vi "Actor Core.vi"(8 "error in":errorcluster, 11 "Post Analysis in":refnum<class "Post Analysis.lvclass">) -> (0 "error out":errorcluster, 3 "Actor out":refnum<class "Actor.lvclass">)   [LabVIEW 2023, in "Data Analysis.lvlib" / "Post Analysis.lvlib" / "Post Analysis.lvclass"]
doc: "(<B>Filename</B>: Actor Framework.lvlib:Actor.lvclass:Actor Core.vi)\n\nReceives messages to the actor, reacts to them, and initiates any error handling that may shut the actor down.\n\nDescendant classes may override this VI to append parallel tasks for the actor to complete while it handles messages. Overrides use the Call Parent Class Method node."
uses:
  Post Analysis.lvclass
  Post Analysis.lvclass/Post Analysis.ctl
  <vilib>/ActorFramework/Actor/Actor.lvclass
  Post Analysis Messages/Init App Msg/Init App Msg.lvclass
  Subpanel-Abstract Messages/Close SP Msg/Close SP Msg.lvclass
  Post Analysis Messages/Launcher Nested Actor Caller Msg/Launcher Nested Actor Caller Msg.lvclass
  Post Analysis Messages/Test Schema Selector Update Msg/Test Schema Selector Update Msg.lvclass
  Post Analysis Messages/Report Data Update the Caller Msg/Report Data Update the Caller Msg.lvclass
  Control/Report.ctl
  Data Analysis.lvlib
  Post Analysis Messages/Filter Name Update the Selector Msg/Filter Name Update the Selector Msg.lvclass
  Post Analysis Messages/Filter Data Clear Msg/Filter Data Clear Msg.lvclass
  Post Analysis Messages/Update Test Schema Msg/Update Test Schema Msg.lvclass
  Post Analysis Messages/Delete the Schema Msg/Delete the Schema Msg.lvclass
  C:/Program Files/National Instruments/LabVIEW 2023/vi.lib/ActorFramework/Actor/Actor.lvclass
  Control/SideMenuBar.ctl
panel:
  in  "Test Phase":string(combo)
  in  "Product":string(combo)
  in  "Test Name":string(combo)
  in  "Delete Log":bool
  in  "Refresh Schema":bool
  in  "Reset Filter":bool
  in  "Test Mode":string(combo)
  in  "Stop Test Cycle":string(combo) caption="Test Cycle"
  in  "Start Test Cycle":string(combo) caption="Test Cycle"
  in  "Test Socket":string(combo)
  in  "Frame Type":string(combo)="fe_frame_log"
  in  "Log in And Out":bool
  in  "Menubar":T1(radio)
  in  "Stop":bool
  out "User":string="Coder "
  in  "Menu":bool
  out "Time":string="03:22:21 PM"
  out "Date":string="18/02/2019"
  out "User Level":string="Operator"
  out "Panel Name":string="Test Panel"
  in  "Sidebar":T2
  in  "Test Log":string(combo)
  # "LTT DATA ANALYSER"
  # "to"
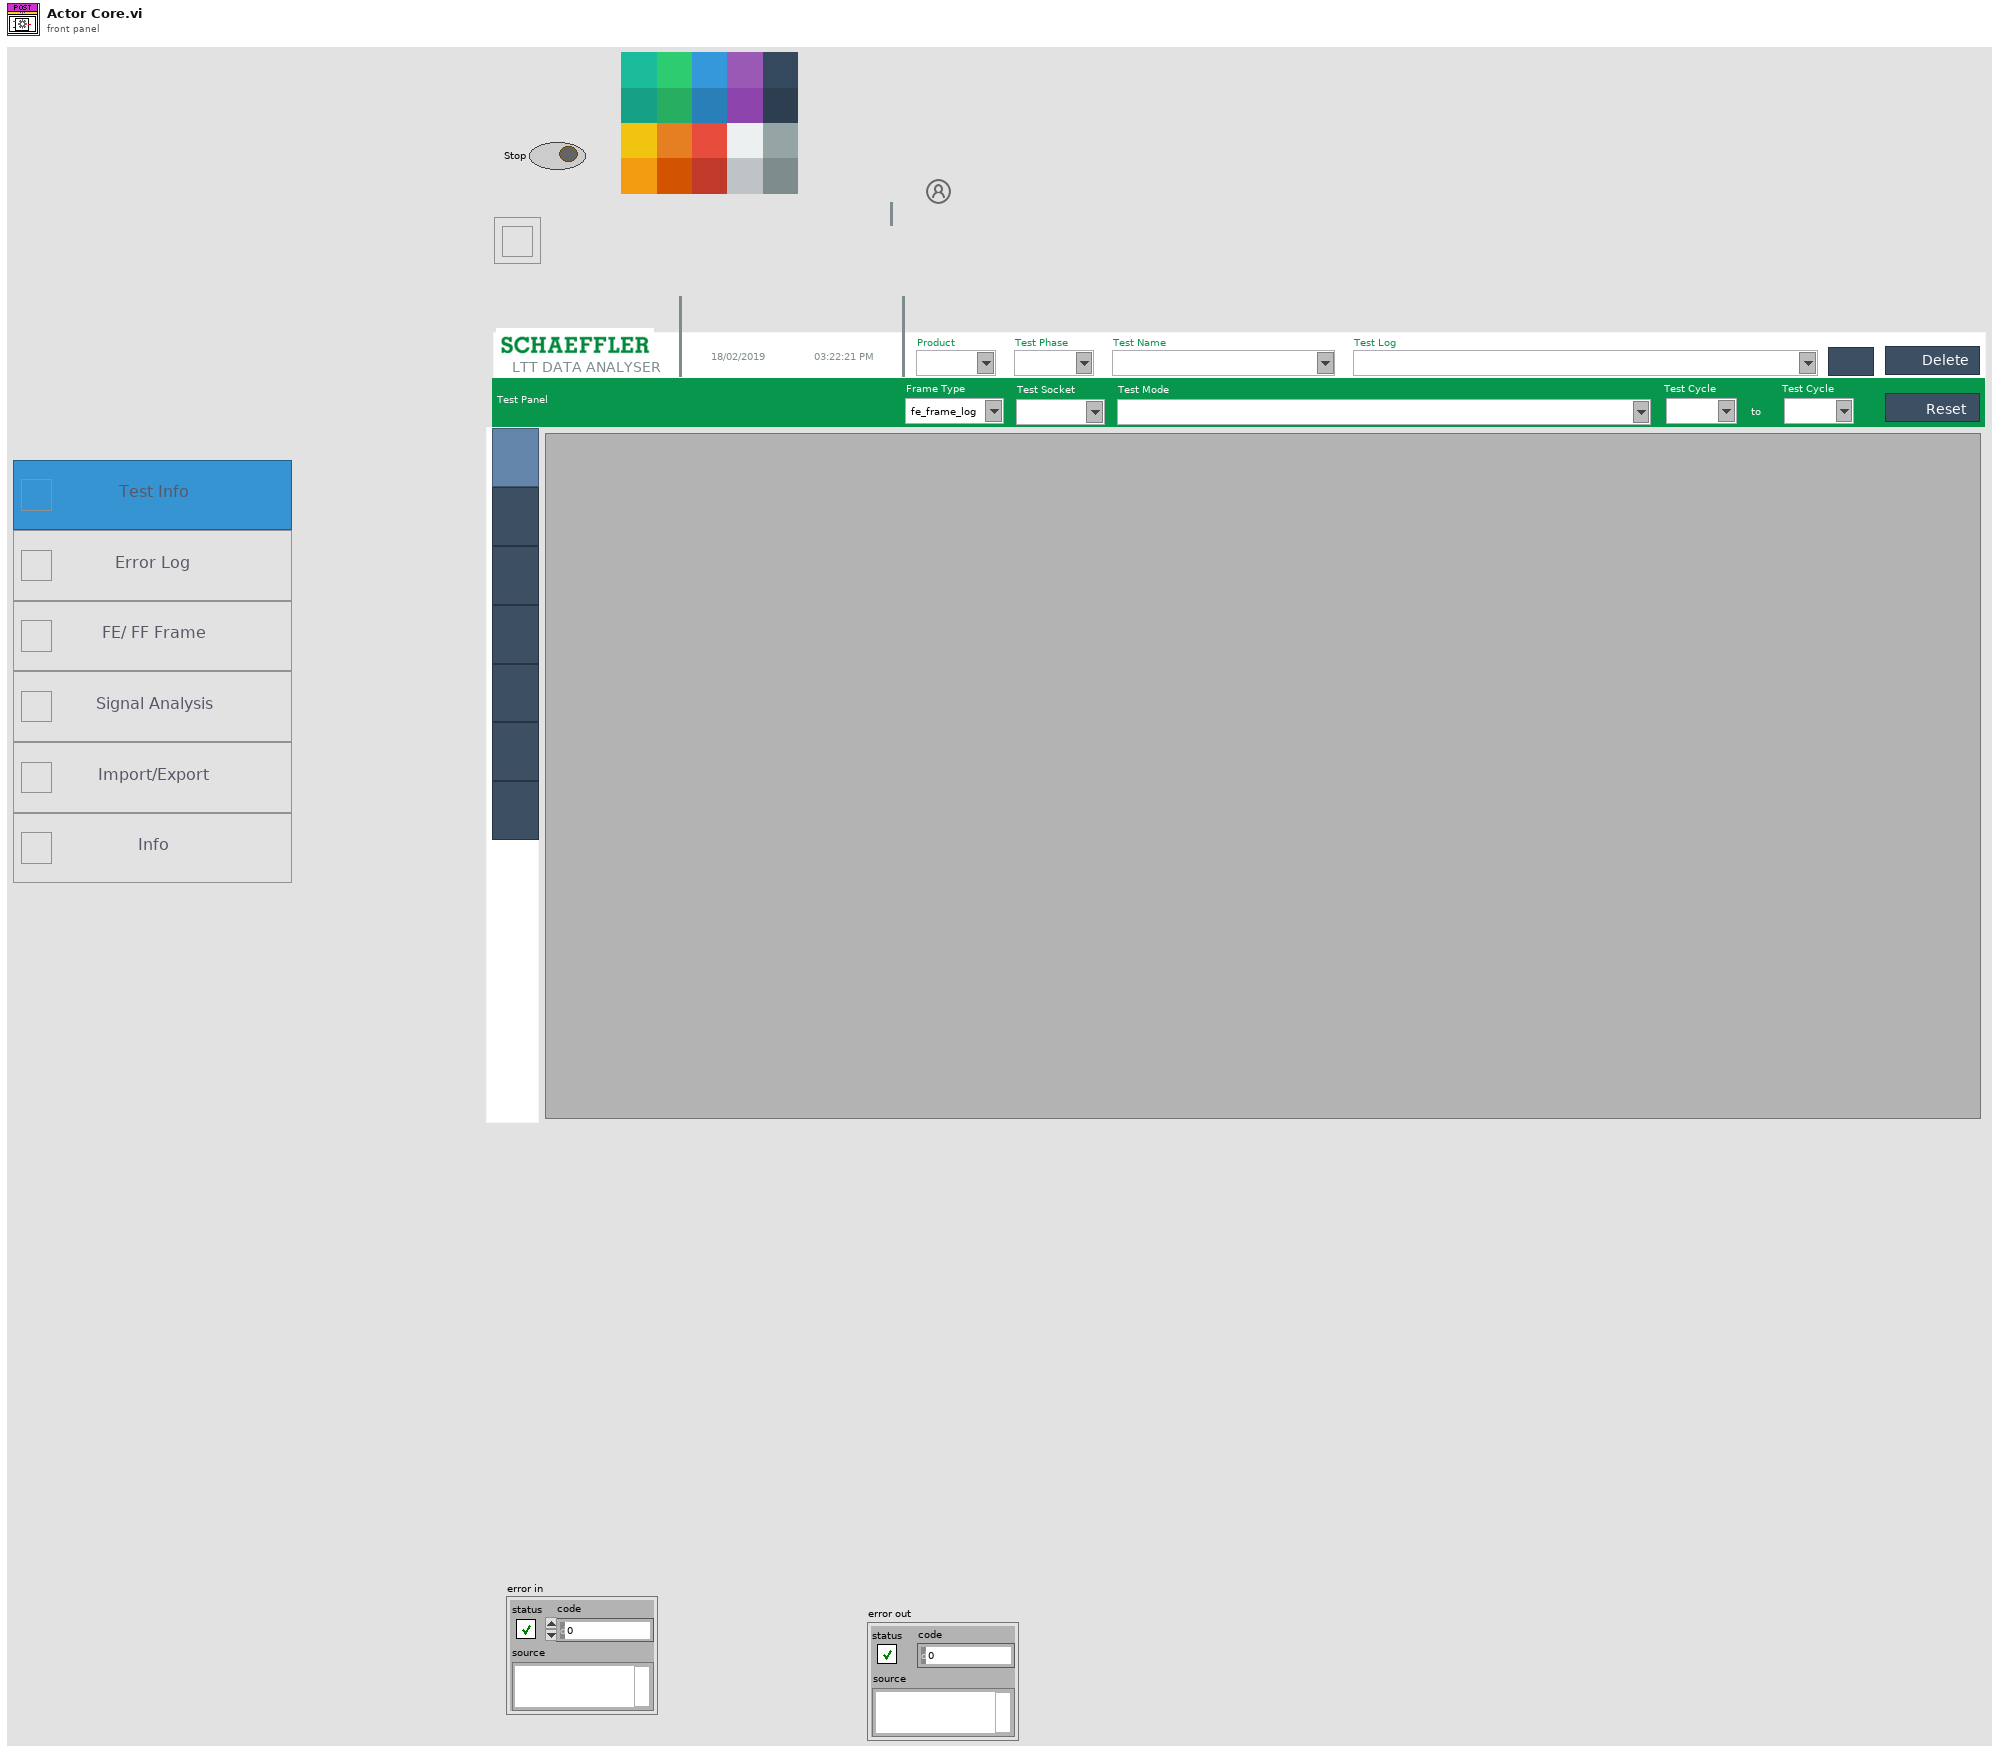
[diagram p1: front panel]
types:
  T1 = enum32{"Test Info", "Error Log", "FE/ FF Frame", "Signal Analysis", "Import/Export", "Info"}
  T2 = typedef "Data Analysis.lvlib/SideMenuBar.ctl" = enum32{"Test Info", "Error Log", "FE/FF Frame", "Signal Analysis", "Export Data", "Test Log Import/Export", "Info"}
  T3 = typedef "Data Analysis.lvlib/Report.ctl" = cluster{"Schema":string, "Test Socket":string, "Start Test Cycle":string, "Stop Test Cycle":string, "Test Mode":string, "Frame Type":string}
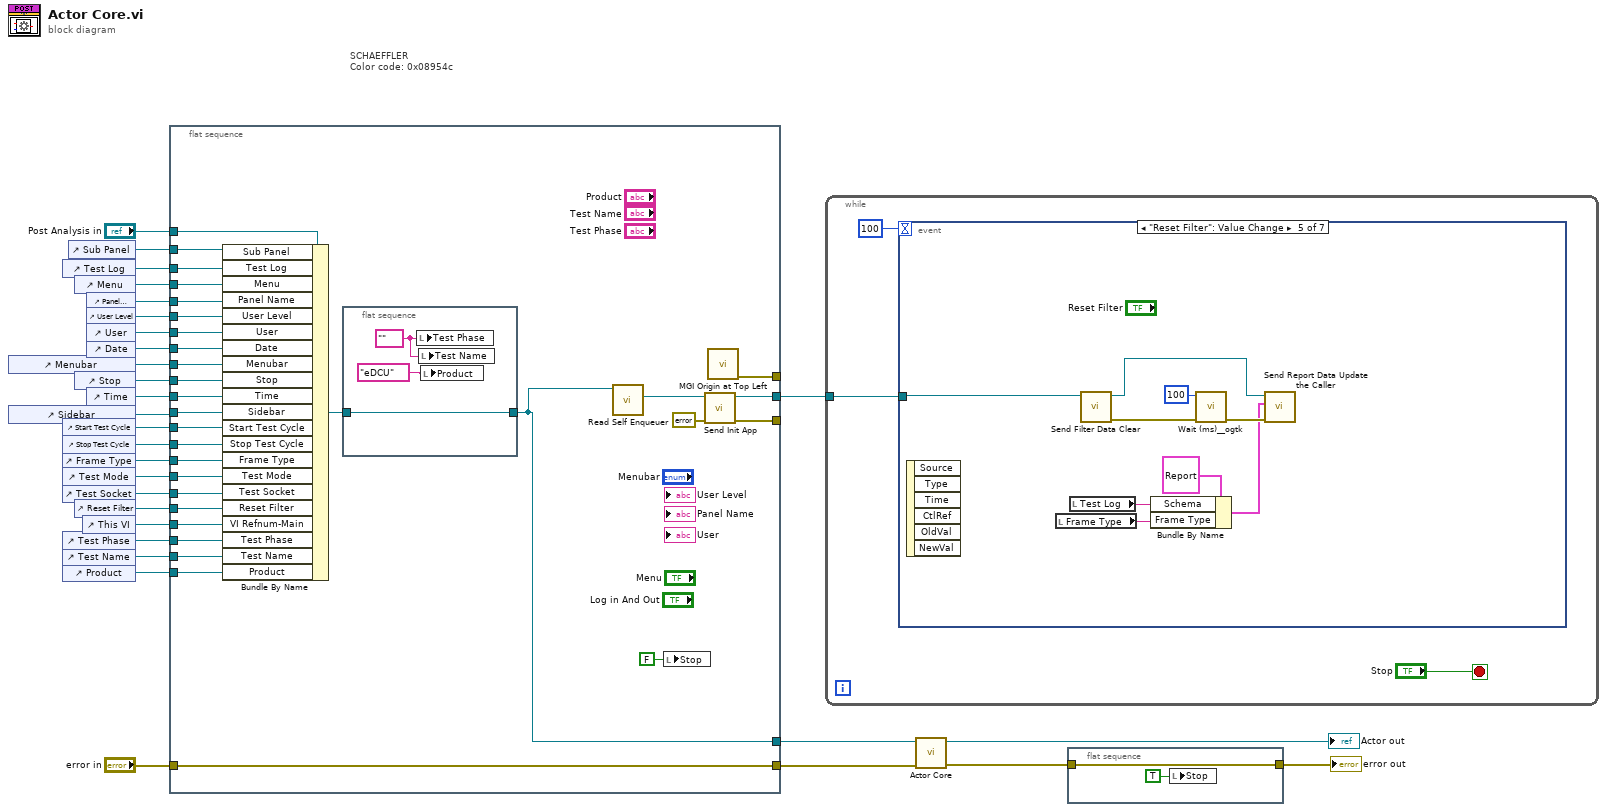
[diagram p0: block diagram]
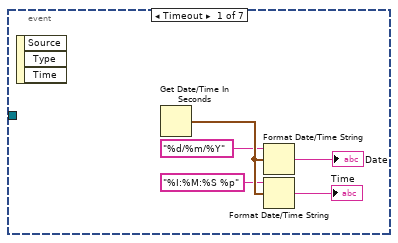
[diagram p2: hidden frame]
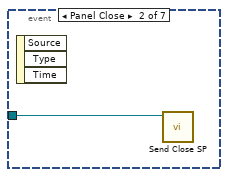
[diagram p3: hidden frame]
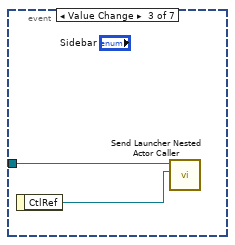
[diagram p4: hidden frame]
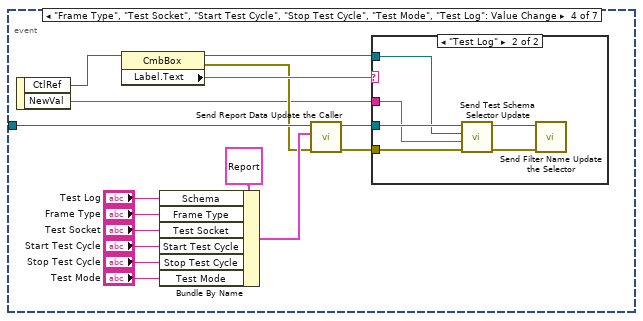
[diagram p5: hidden frame]
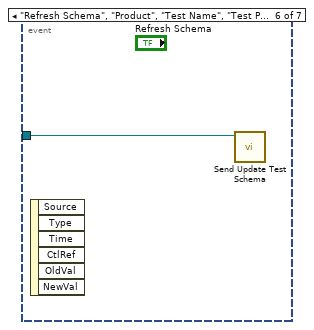
[diagram p7: hidden frame]
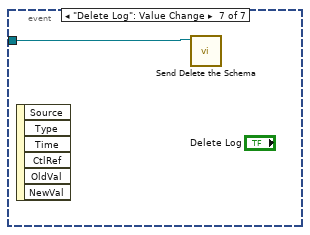
[diagram p8: hidden frame]
diagram:
  # "SCHAEFFLER \nColor code: 0x08954c"
  n1 = control-ref of="Menubar"() -> (w12:refnum<vi>)
  n2 = control-ref of="Sidebar"() -> (w1:refnum<vi>)
  n3 = control-ref of="Test Log"() -> (w23:refnum<vi>)
  n4 = control-ref of="Start Test Cycle"() -> (w11:refnum<vi>)
  n5 = control-ref of="Stop Test Cycle"() -> (w10:refnum<vi>)
  n6 = control-ref of="Frame Type"() -> (w9:refnum<vi>)
  n7 = control-ref of="Test Mode"() -> (w8:refnum<vi>)
  n8 = control-ref of="Test Socket"() -> (w7:refnum<vi>)
  n9 = control-ref of="Test Phase"() -> (w4:refnum<vi>)
  n10 = control-ref of="Test Name"() -> (w3:refnum<vi>)
  n11 = control-ref of="Product"() -> (w2:refnum<vi>)
  n12 = control-ref of="Sub Panel"() -> (w24:refnum<vi>)
  n13 = control-ref of="Menu"() -> (w22:refnum<vi>)
  n14 = control-ref of="Stop"() -> (w17:refnum<vi>)
  n15 = control-ref of="Reset Filter"() -> (w6:refnum<vi>)
  n16 = control-ref of="This VI"() -> (w5:refnum<vi>)
  n17 = control-ref of="Panel Name"() -> (w21:refnum<vi>)
  n18 = control-ref of="User Level"() -> (w20:refnum<vi>)
  n19 = control-ref of="User"() -> (w19:refnum<vi>)
  n20 = control-ref of="Date"() -> (w18:refnum<vi>)
  n21 = control-ref of="Time"() -> (w16:refnum<vi>)
  n22 = flat-sequence {
    tunnel: "Post Analysis in" -> [w56]
    tunnel: [w31] -> w28
    tunnel: "error in" -> [w60]
    tunnel: [w60] -> w26
    tunnel: [w59] -> _
    tunnel: [w57] -> w25
    tunnel: w24 -> [w55]
    tunnel: w23 -> [w54]
    tunnel: w22 -> [w53]
    tunnel: w21 -> [w52]
    tunnel: w20 -> [w51]
    tunnel: w19 -> [w50]
    tunnel: w18 -> [w49]
    tunnel: w17 -> [w48]
    tunnel: w16 -> [w47]
    tunnel: w1 -> [w30]
    tunnel: w12 -> [w45]
    tunnel: w11 -> [w44]
    tunnel: w10 -> [w43]
    tunnel: w9 -> [w42]
    tunnel: w8 -> [w41]
    tunnel: w7 -> [w40]
    tunnel: [w38] -> _
    tunnel: w6 -> [w37]
    tunnel: w5 -> [w36]
    tunnel: w4 -> [w35]
    tunnel: w3 -> [w34]
    tunnel: w2 -> [w33]
    frame #0 {
      n23 = Bundle By Name(cluster=w56, "Sub Panel"=w55, "Test Log"=w54, "Menu"=w53, "Panel Name"=w52, "User Level"=w51, "User"=w50, "Date"=w49, "Menubar"=w45, "Stop"=w48, "Time"=w47, "Sidebar"=w30, "Start Test Cycle"=w44, "Stop Test Cycle"=w43, "Frame Type"=w42, "Test Mode"=w41, "Test Socket"=w40, "Reset Filter"=w37, "VI Refnum-Main"=w36, "Test Phase"=w35, "Test Name"=w34, "Product"=w33) -> (w32:refnum<class "Post Analysis.lvclass">)
      n24 = flat-sequence {
        tunnel: [w61] -> w31
        tunnel: w32 -> [w61]
        frame #0 {
          w63 = "" ("Test Phase")
          n25 = local write "Test Phase"(w63) -> ()
          n26 = local write "Test Name"(w63) -> ()
          n27 = local write "Product"("eDCU" ("Product")) -> ()
        }
      }
      n28 = call <vilib>:"Read Self Enqueuer.vi"("Actor"=w31) -> ("Self Enqueuer"=w58:refnum<class "Message Enqueuer.lvclass">)  [unwired: 10 in]
      n29 = local write "Stop"(FALSE ("Stop")) -> ()
      n30 = call "Send Init App.vi"("error in (no error)"=errorcluster {"status"=FALSE, "code"=0, "source"=""}, "Message Enqueuer"=w58) -> ("error out"=w38:errorcluster, "Message Enqueuer out"=w57:refnum<class "Message Enqueuer.lvclass">)  [unwired: 8 in]
      n31 = call <userlib>:"MGI Origin at Top Left.vi"() -> ("Error Out"=w59:errorcluster)  [unwired: 9 in, 1 out]
    }
  }
  n32 = while {
    tunnel: w25 -> [w65]
    stop <- "Stop" stop-if-true
    n33 = event shown="[4] \"Reset Filter\": Value Change" {
      selector: _ -> [_ _ _ _ _ _ _]
      dyn-events: _ -> [_ _ _ _ _ _ _]
      timeout: 100 -> [_ _ _ _ _ _ _]
      tunnel: w65 -> [_ w72 w74 w90 w105 w106 w107]
      event Timeout {
        n34 = event-data() -> ()  [unwired: 1 in, 3 out]
        n35 = Get Date/Time In Seconds() -> (seconds since 1Jan1904=w71:timestamp)
        n36 = Format Date/Time String(time format string (%c)="%d/%m/%Y", seconds (now)=w71) -> (date/time string=→"Date":string)  [unwired: 1 in]
        n37 = Format Date/Time String(time format string (%c)="%I:%M:%S %p", seconds (now)=w71) -> (date/time string=→"Time":string)  [unwired: 1 in]
      }
      event Panel Close {
        n38 = event-data() -> ()  [unwired: 1 in, 3 out]
        n39 = call "Send Close SP.vi"("Message Enqueuer"=w72) -> ()  [unwired: 9 in, 2 out]
      }
      event Value Change {
        n40 = event-data() -> ("CtlRef"=w73:refnum<vi>)  [unwired: 1 in]
        n41 = call "Send Launcher Nested Actor Caller.vi"("Sidebar"=w73, "Message Enqueuer"=w74) -> ()  [unwired: 8 in, 2 out]
      }
      event "Frame Type", "Test Socket", "Start Test Cycle", "Stop Test Cycle", "Test Mode", "Test Log": Value Change {
        n42 = event-data() -> ("CtlRef"=w81:refnum<vi>, "NewVal"=w75:string)  [unwired: 1 in]
        n43 = property class="CmbBox"(reference=w81) -> (reference out=w78:refnum<vi>, error out=w76:errorcluster, "Label.Text"=w77:string)  [unwired: 1 in]
        n44 = Bundle By Name(cluster=T3 {"Schema"="", "Test Socket"="", "Start Test Cycle"="", "Stop Test Cycle"="", "Test Mode"="", "Frame Type"="fe_frame_log"} ("Report Data"), "Schema"="Test Log", "Frame Type"="Frame Type", "Test Socket"="Test Socket", "Start Test Cycle"="Start Test Cycle", "Stop Test Cycle"="Stop Test Cycle", "Test Mode"="Test Mode") -> (w82:T3)
        n45 = call "Send Report Data Update the Caller.vi"("error in (no error)"=w76, "Report Data"=w82, "Message Enqueuer"=w90) -> ("error out"=w80:errorcluster, "Message Enqueuer out"=w79:refnum<class "Message Enqueuer.lvclass">)  [unwired: 7 in]
        n46 = case shown="\"Test Log\"" w77 {
          tunnel: w80 -> [_ w94]
          tunnel: w79 -> [_ w93]
          tunnel: w78 -> [_ w92]
          tunnel: w75 -> [_ w91]
          frame Default {
          }
          frame "Test Log" {
            n47 = call "Send Test Schema Selector Update.vi"("error in (no error)"=w94, "Schema"=w91, "Test Log"=w92, "Message Enqueuer"=w93) -> ("error out"=w95:errorcluster, "Message Enqueuer out"=w96:refnum<class "Message Enqueuer.lvclass">)  [unwired: 6 in]
            n48 = call "Send Filter Name Update the Selector.vi"("error in (no error)"=w95, "Message Enqueuer"=w96) -> ()  [unwired: 8 in, 2 out]
          }
        }
      }
      event "Reset Filter": Value Change {
        n49 = event-data() -> ()  [unwired: 1 in, 6 out]
        n50 = local read "Frame Type"() -> (w97:string)
        n51 = local read "Test Log"() -> (w98:string)
        n52 = call "Send Filter Data Clear.vi"("Message Enqueuer"=w105) -> ("error out"=w103:errorcluster, "Message Enqueuer out"=w99:refnum<class "Message Enqueuer.lvclass">)  [unwired: 9 in]
        n53 = Bundle By Name(cluster=T3 {"Schema"="", "Test Socket"="", "Start Test Cycle"="", "Stop Test Cycle"="", "Test Mode"="", "Frame Type"="fe_frame_log"} ("Report Data"), "Schema"=w98, "Frame Type"=w97) -> (w100:T3)
        n54 = call <userlib>:"Wait (ms)__ogtk.vi"("error in (no error)"=w103, "milliseconds to wait"=u32 100) -> ("error out"=w101:errorcluster)  [unwired: 8 in, 1 out]
        n55 = call "Send Report Data Update the Caller.vi"("error in (no error)"=w101, "Report Data"=w100, "Message Enqueuer"=w99) -> ()  [unwired: 7 in, 2 out]
      }
      event "Refresh Schema", "Product", "Test Name", "Test Phase": Value Change {
        n56 = event-data() -> ()  [unwired: 1 in, 6 out]
        n57 = call "Send Update Test Schema.vi"("Message Enqueuer"=w106) -> ()  [unwired: 9 in, 2 out]
      }
      event "Delete Log": Value Change {
        n58 = event-data() -> ()  [unwired: 1 in, 6 out]
        n59 = call "Send Delete the Schema.vi"("Message Enqueuer"=w107) -> ()  [unwired: 9 in, 2 out]
      }
    }
  }
  n60 = call-parent "Actor Core.vi"("error in"=w26, "Actor in"=w28) -> ("error out"=w14:errorcluster, "Actor out"=→"Actor out":refnum<class "Actor.lvclass">)  [unwired: 8 in]
  n61 = flat-sequence {
    tunnel: w14 -> [w109]
    tunnel: [w109] -> w13
    frame #0 {
      n62 = local write "Stop"(TRUE ("Stop")) -> ()
    }
  }
  "error out" <- w13
